vi "PC_Pub_imgFile checkPropertyValid.vi"(8 "error in (no error)":errorcluster, 11 "imgFile in":refnum<class "PC_Pub_imgFile.lvclass">) -> (0 "error out":errorcluster, 1 "appended path":path, 2 "Image Metadata in":T1={"title"="", "description"="", "ID"="", "version"="", "component type"=5} caption="Image Metadata out" {"component type" items=["standard", "hidden", "system", "unknown", "startup", "image"]}, 3 "imgFile out":refnum<class "PC_Pub_imgFile.lvclass">, 4 "valid":bool)   [LabVIEW 2018, in "PC_Pub_imgFile.lvclass"]
uses:
  PC_Pub_imgFile.lvclass
  <vilib>/nisyscfg/Software 1.2.ctl
  <vilib>/nisyscfg/Component Type.ctl
  PC_Pub_imgFile.lvclass/PC_Pub_imgFile.ctl
  <vilib>/nisyscfg/nisyscfg.lvlib
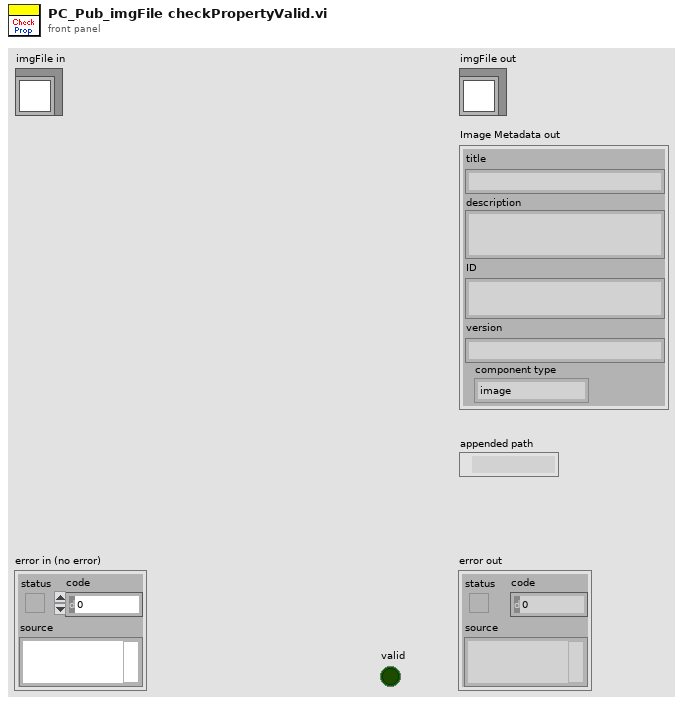
[diagram p1: front panel]
types:
  T1 = typedef "nisyscfg.lvlib/Software 1.2.ctl" = cluster{"title":string, "description":string, "ID":string, "version":string, "component type":T2}
  T2 = typedef "nisyscfg.lvlib/Component Type.ctl" = u32
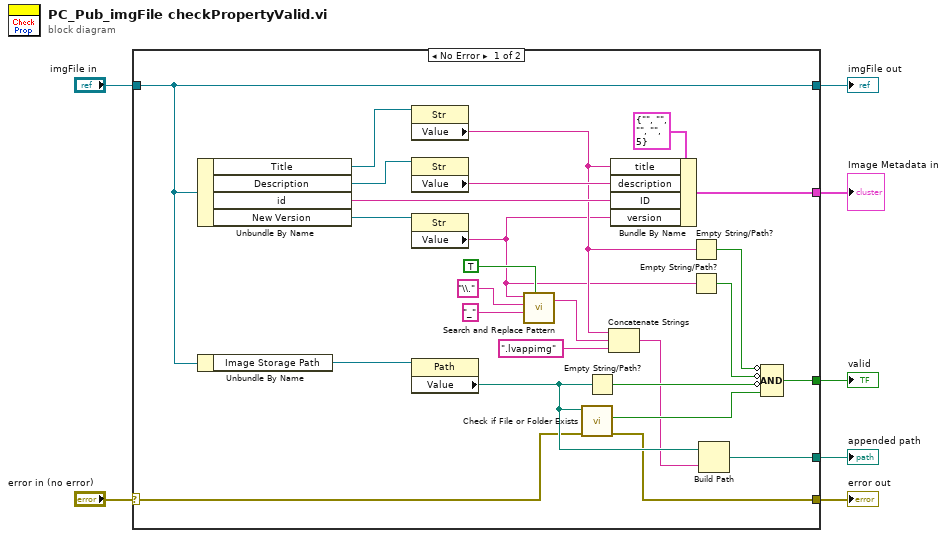
[diagram p0: block diagram]
diagram:
  n1 = case shown="No Error" "error in (no error)" {
    selector: "error in (no error)" -> [w10 w35]
    tunnel: [w8 w35] -> w6
    tunnel: [w17 w34] -> w4
    tunnel: "imgFile in" -> [w17 w34]
    tunnel: [w31 _] -> w3
    tunnel: [w11 _] -> w2
    tunnel: [w9 _] -> w1
    frame No Error {
      n2 = Unbundle By Name(w17) -> ("Title"=w29:refnum<vi>, "Description"=w28:refnum<vi>, "id"=w26:string, "New Version"=w27:refnum<vi>)
      n3 = Unbundle By Name(w17) -> ("Image Storage Path"=w16:refnum<vi>)
      n4 = property class="Str"(reference=w29) -> ("Value"=w19:string)  [unwired: 1 in, 2 out]
      n5 = property class="Str"(reference=w28) -> ("Value"=w25:string)  [unwired: 1 in, 2 out]
      n6 = property class="Str"(reference=w27) -> ("Value"=w18:string)  [unwired: 1 in, 2 out]
      n7 = property class="Path"(reference=w16) -> ("Value"=w13:path)  [unwired: 1 in, 2 out]
      n8 = call <vilib>:"Search and Replace Pattern.vi"("string"=w18, "regular expression (\"\")"="\\." ("regular expression (\"\")"), "replace string (\"\")"="_" ("replace string (\"\")"), "replace all? (F)"=TRUE) -> ("result string"=w21:string)  [unwired: 1 in, 1 out]
      n9 = call <vilib>:"Check if File or Folder Exists.vi"("error in (no error)"=w10, "path"=w13) -> ("error out"=w8:errorcluster, "file or folder exists?"=w14:bool)  [unwired: 7 in, 1 out]
      n10 = Empty String/Path?(string/path=w13) -> (empty?=w15:bool)
      n11 = Concatenate Strings(w19, w21, ".lvappimg" ("string")) -> (w12:string)
      n12 = Bundle By Name(cluster=T1 {"title"="", "description"="", "ID"="", "version"="", "component type"=5} ("Image Metadata in"), "title"=w19, "description"=w25, "ID"=w26, "version"=w18) -> (w11:T1)
      n13 = Empty String/Path?(string/path=w19) -> (empty?=w33:bool)
      n14 = Empty String/Path?(string/path=w18) -> (empty?=w32:bool)
      n15 = Build Path(base path=w13, name or relative path=w12) -> (appended path=w9:path)
      n16 = Compound Arithmetic op=AND(invert w33, invert w32, invert w15, w14) -> (w31:bool)
    }
    frame Error {
    }
  }
  "error out" <- w6
  "imgFile out" <- w4
  "valid" <- w3
  "Image Metadata in" <- w2
  "appended path" <- w1
